vi "FWHM2.vi"(0 "Input X":dbl[](array[numeric]), 1 "Inpput Y":dbl[](array[numeric])) -> (2 "FWHM in X":dbl, 3 "dE/E":dbl, 4 "X Peak location":dbl)   [LabVIEW 2013]
panel:
  out "FWHM (array-min(array))":dbl
  out "FWHM in index":dbl
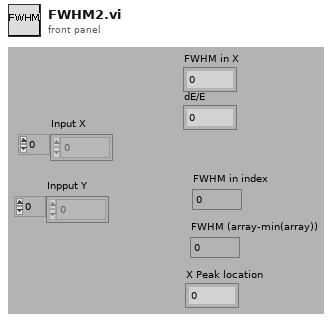
[diagram p1: front panel]
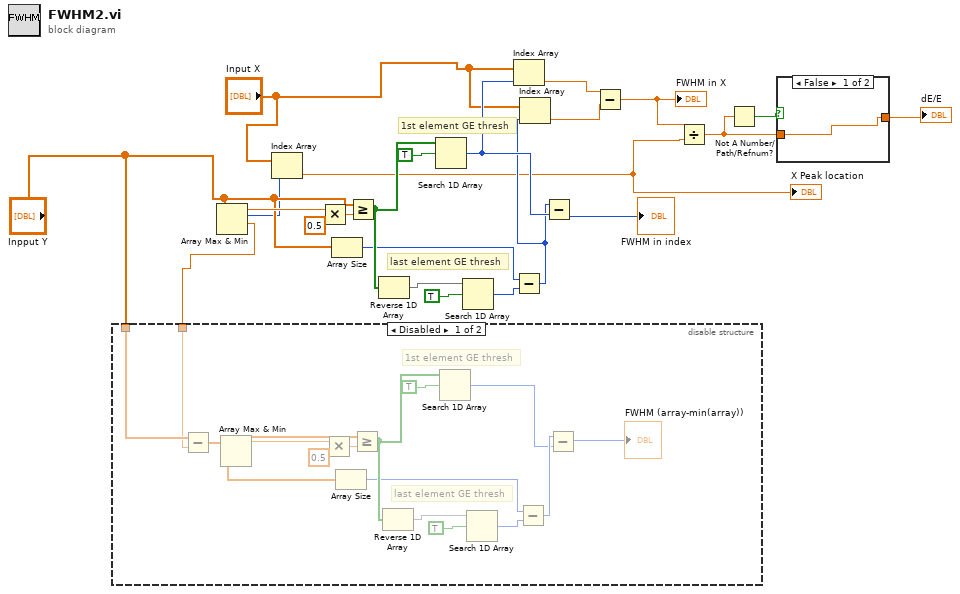
[diagram p0: block diagram]
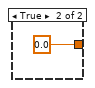
[diagram p2: hidden frame]
diagram:
  # "last element GE thresh"
  # "1st element GE thresh"
  n1 = Array Max & Min(array="Inpput Y") -> (max value=w21:dbl, max index (indices)=w6:i32, min value=w12:dbl)  [unwired: 1 out]
  n2 = disable-structure shown="Disabled" {
    disable-tunnel: "Inpput Y" -> [w25 _]
    disable-tunnel: w12 -> [w24 _]
    frame Disabled {
      # "last element GE thresh"
      # "1st element GE thresh"
      n3 = Subtract(x=w25, y=w24) -> (x-y=w29:dbl[])
      n4 = Array Max & Min(array=w29) -> (max value=w36:dbl)  [unwired: 3 out]
      n5 = Multiply(x=w36, y=0.5) -> (x*y=w38:dbl)
      n6 = Array Size(array=w29) -> (size(s)=w31:i32)
      n7 = Greater Or Equal?(x=w29, y=w38) -> (x >= y?=w34:bool[])
      n8 = Reverse 1D Array(array=w34) -> (reversed array=w32:bool[])
      n9 = Search 1D Array(1D array=w34, element=TRUE) -> (index of element=w26:i32)  [unwired: 1 in]
      n10 = Search 1D Array(1D array=w32, element=TRUE) -> (index of element=w30:i32)  [unwired: 1 in]
      n11 = Subtract(x=w31, y=w30) -> (x-y=w27:i32)
      n12 = Subtract(x=w27, y=w26) -> (x-y=→"FWHM (array-min(array))":i32)
    }
    frame Enabled {
    }
  }
  n13 = Index Array(array="Input X", index=w6) -> (element=w4:dbl)
  "X Peak location" <- w4
  n14 = Multiply(x=w21, y=0.5) -> (x*y=w23:dbl)
  n15 = Array Size(array="Inpput Y") -> (size(s)=w16:i32)
  n16 = Greater Or Equal?(x="Inpput Y", y=w23) -> (x >= y?=w19:bool[])
  n17 = Reverse 1D Array(array=w19) -> (reversed array=w17:bool[])
  n18 = Search 1D Array(1D array=w19, element=TRUE) -> (index of element=w11:i32)  [unwired: 1 in]
  n19 = Search 1D Array(1D array=w17, element=TRUE) -> (index of element=w15:i32)  [unwired: 1 in]
  n20 = Index Array(array="Input X", index=w11) -> (element=w8:dbl)
  n21 = Subtract(x=w16, y=w15) -> (x-y=w10:i32)
  n22 = Index Array(array="Input X", index=w10) -> (element=w9:dbl)
  n23 = Subtract(x=w10, y=w11) -> (x-y=→"FWHM in index":i32)
  n24 = Subtract(x=w8, y=w9) -> (x-y=w5:dbl)
  "FWHM in X" <- w5
  n25 = Divide(x=w5, y=w4) -> (x/y=w1:dbl)
  n26 = Not A Number/Path/Refnum?(number/path/refnum=w1) -> (NaN/Path/Refnum?=w3:bool)
  n27 = case shown="False" w3 {
    tunnel: [w39 0.0] -> w2
    tunnel: w1 -> [w39 _]
    frame False {
    }
    frame True {
    }
  }
  "dE/E" <- w2
